vi "ObtainResult.vi"(8 "ErrorIn":errorcluster, 9 "DefaultResult":refnum<class "IResult.lvclass">, 10 "Name":string, 11 "TopModuleIn":refnum<class "TopModule.lvclass">) -> (0 "ErrorOut":errorcluster, 1 "ResultOut":refnum<class "IResult.lvclass">, 2 "Result Not Found?":bool, 3 "TopModuleOut":refnum<class "TopModule.lvclass">)   [LabVIEW 2019, in "TopModule.lvclass"]
uses:
  TopModule.lvclass
  IResult/IResult.lvclass
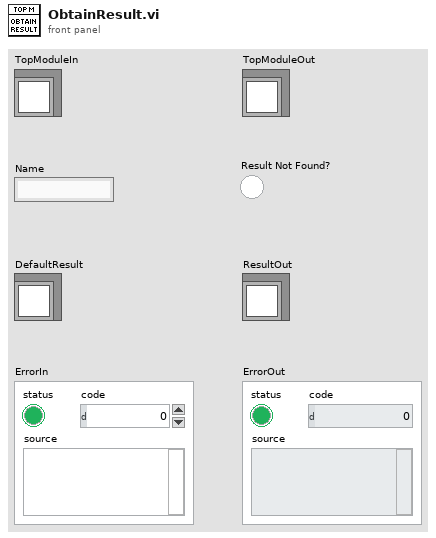
[diagram p1: front panel]
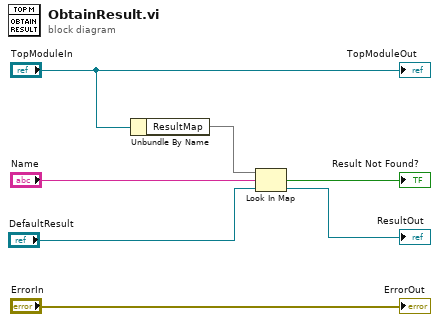
[diagram p0: block diagram]
diagram:
  n1 = Unbundle By Name("TopModuleIn") -> ("ResultMap"=w6:map{string, refnum<class "IResult.lvclass">})
  n2 = Look In Map(map=w6, key="Name", default value="DefaultResult") -> (key not found?=→"Result Not Found?":bool, value=→"ResultOut":refnum<class "IResult.lvclass">)
  "TopModuleOut" <- "TopModuleIn"
  "ErrorOut" <- "ErrorIn"
